vi "P116x1ch_WriteManual.vi"(5 "P116x1ch":T1, 7 "Decimales":T3=1 items=["0"=1, "1"=10, "2"=100], 8 "error in (no error)":errorcluster, 9 "RateSP":T2, 10 "NuevoSP":T2, 11 "Comunicaciones":T4={"Eurotherm"="ASRL6::INSTR", "CDT"=FALSE, "Agilent"="ASRL6::INSTR", "AGL"=FALSE, "#dec"=1} {"#dec" items=["1"=1, "1"=10, "2"=100]}) -> (0 "error out":errorcluster, 1 "RateSP(C/min) 2":T2, 2 "NuevoSP(C) 2":T2)   [LabVIEW 2017]
uses:
  1xP116.ctl
  Typedefs/SECADO_comms--Cluster.ctl
  numDecimales--Enum.ctl
  P116x1ch.ctl
  Address.ctl
  Eurotherm_2023_Module.ctl
panel:
  out "PV":T2
  out "WorkingSP":T2
  out "TargetSP":T2
  in  "Cancel":bool
  in  "Write":bool
  out "Enable(T)":bool=TRUE
  out "VISA Promux":refnum<visa-resource-name>
  in  "Delay Time (s)":dbl=0.1
  # "Programando Eurotherm"
  # "C/min"
  # "C"
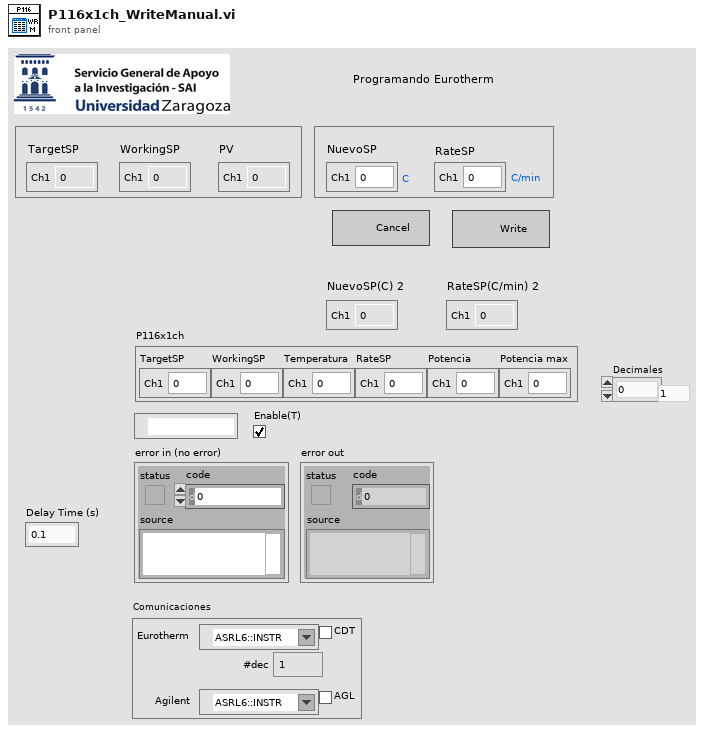
[diagram p1: front panel]
types:
  T1 = typedef "P116x1ch.ctl" = cluster{"TargetSP":T2, "WorkingSP":T2, "Temperatura":T2, "RateSP":T2, "Potencia":T2, "Potencia max":T2}
  T2 = typedef "1xP116.ctl" = cluster{"Ch1":dbl}
  T3 = typedef "numDecimales--Enum.ctl" = u16
  T4 = typedef "SECADO_comms--Cluster.ctl" = cluster{"Eurotherm":refnum<visa-resource-name>, "CDT":bool, "Agilent":refnum<visa-resource-name>, "AGL":bool, "#dec":T3}
  T5 = typedef "Eurotherm_2023_Module.ctl" = enum16{"Initialize", "Write setpoint", "Read data", "Write ramp rate", "Set constante proporcional", "Set constante integral", "Set constante diferencial", "Set ouput limit LOW", "Set ouput limit HIGH", "Shutdown"}
  T6 = typedef "Address.ctl" = enum16{"Add 1", "Add 2", "Add 3", "Add 4", "Add 5", "Add 6", "Add 10", "Add 11", "Add 12", "Add 13"}
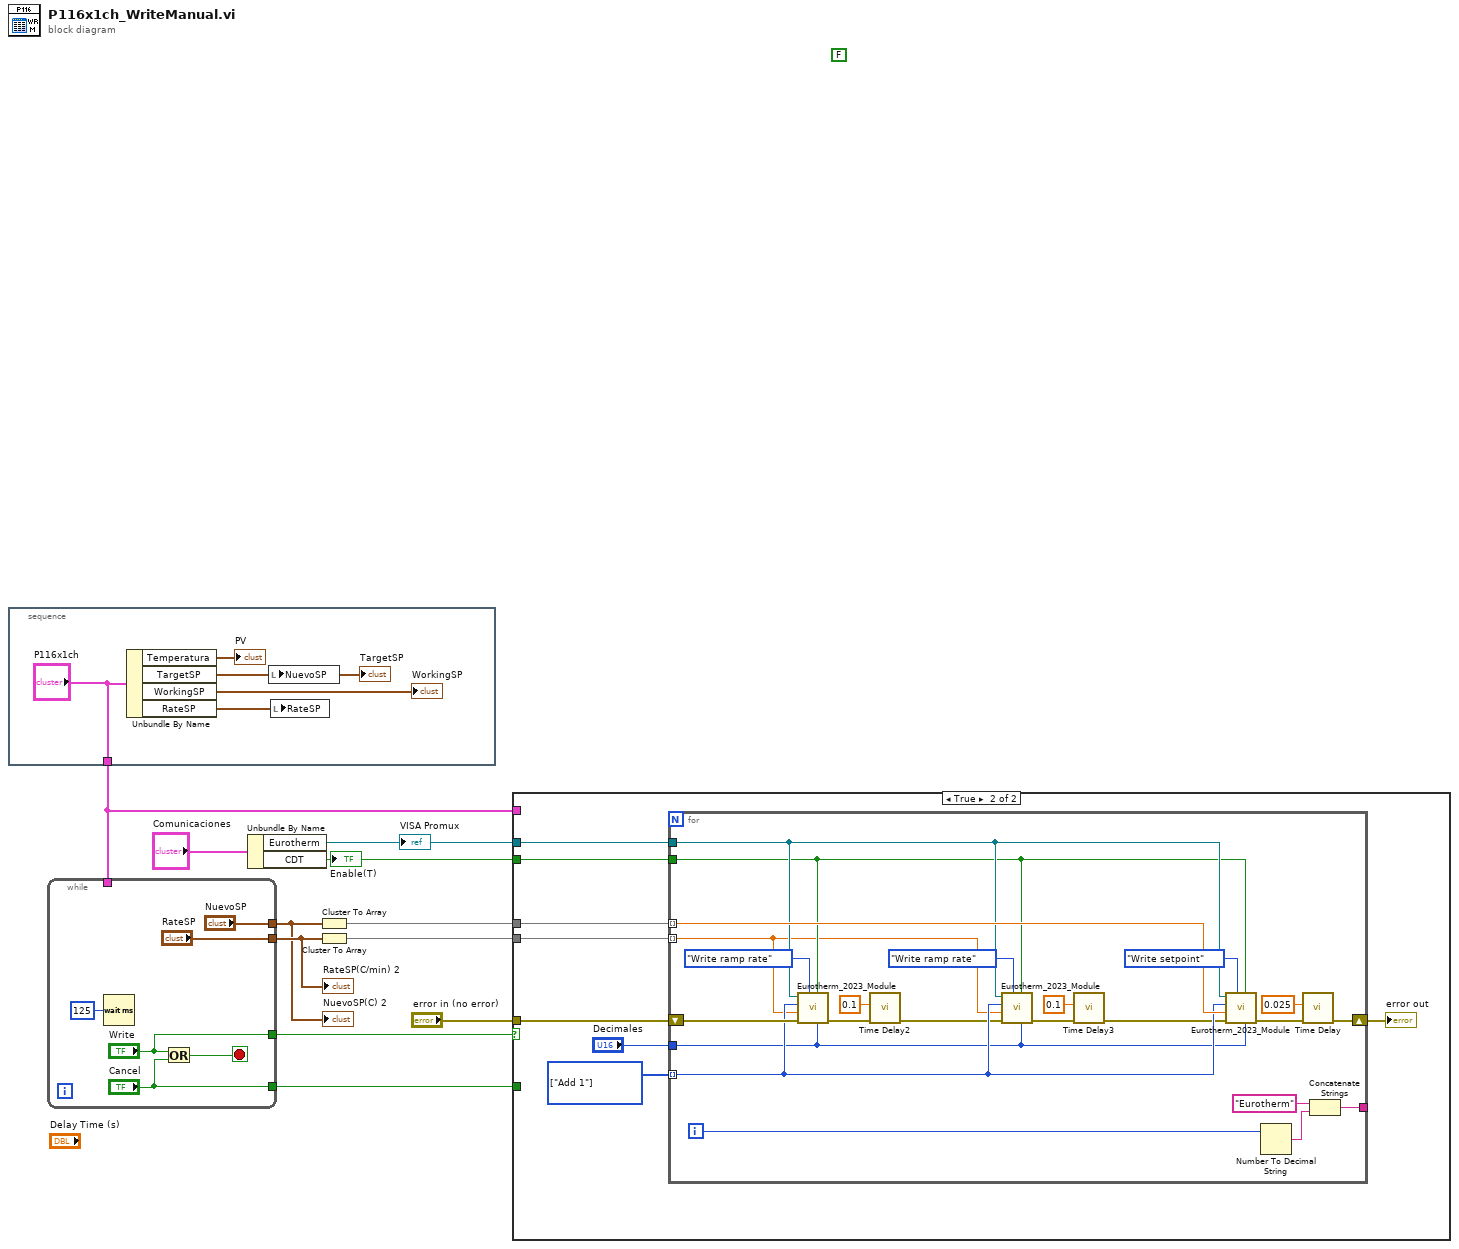
[diagram p0: block diagram]
diagram:
  (unwired) FALSE
  n1 = stacked-sequence {
    tunnel: ["P116x1ch"] -> w4
    frame #0 {
      n2 = Unbundle By Name("P116x1ch") -> ("Temperatura"=→"PV":T2, "TargetSP"=w14:T2, "WorkingSP"=→"WorkingSP":T2, "RateSP"=w13:T2)
      "TargetSP" <- w14
      n3 = local write "NuevoSP"(w14) -> ()
      n4 = local write "RateSP"(w13) -> ()
    }
  }
  n5 = while {
    tunnel: ["Cancel"] -> w10
    tunnel: ["NuevoSP"] -> w2
    tunnel: ["RateSP"] -> w3
    tunnel: ["Write"] -> w6
    tunnel: w4 -> [_]
    stop <- w17 stop-if-true
    n6 = Wait (ms)(milliseconds to wait=u32 125) -> ()  [unwired: 1 out]
    n7 = Or(x="Write", y="Cancel") -> (x .or. y?=w17:bool)
  }
  "NuevoSP(C) 2" <- w2
  "RateSP(C/min) 2" <- w3
  n8 = Unbundle By Name("Comunicaciones") -> ("Eurotherm"=w5:refnum<visa-resource-name>, "CDT"=w11:bool)
  "Enable(T)" <- w11
  "VISA Promux" <- w5
  n9 = Cluster To Array(cluster=w2) -> (array=w8:dbl[])
  n10 = Cluster To Array(cluster=w3) -> (array=w7:dbl[])
  n11 = case shown="True" w6 {
    tunnel: w11 -> [_ w29]
    tunnel: w10 -> [_ _]
    tunnel: "error in (no error)" -> [_ w27]
    tunnel: w8 -> [_ w25]
    tunnel: w7 -> [_ w26]
    tunnel: w5 -> [_ w30]
    tunnel: w4 -> [_ _]
    frame False {
    }
    frame True {
      w24 = T6[] [enum."Add 1"] items=["Add 1", "Add 2", "Add 3", "Add 4", "Add 5", "Add 6", "Add 10", "Add 11", "Add 12", "Add 13"]
      n12 = for {
        tunnel: w24 -> [w37] mode=indexing
        shift-right: [w44] -> w28
        shift-left: w27 -> [w48]
        tunnel: [w51] -> _
        tunnel: w25 -> [w46] mode=indexing
        tunnel: w26 -> [w32] mode=indexing
        tunnel: w30 -> [w34]
        tunnel: w29 -> [w33]
        tunnel: "Decimales" -> [w31]
        i -> [w43]
        n13 = call "Eurotherm_2023_Module.vi"("Decimales"=w31, "Eurotherm (T:Enable)"=w33, "Command"=Eurotherm_2023_Module."Write ramp rate", "error in (no error)"=w48, "Value"=w32, "Address"=w37, "VISA resource name"=w34) -> ("error out"=w42:errorcluster)  [unwired: 2 in, 2 out]
        n14 = call "Time Delay2"("error in (no error)"=w42, "Delay Time (s)"=0.1) -> ("error out"=w36:errorcluster)  [unwired: 9 in]
        n15 = call "Eurotherm_2023_Module.vi"("Decimales"=w31, "Eurotherm (T:Enable)"=w33, "Command"=Eurotherm_2023_Module."Write ramp rate", "error in (no error)"=w36, "Value"=w32, "Address"=w37, "VISA resource name"=w34) -> ("error out"=w39:errorcluster)  [unwired: 2 in, 2 out]
        n16 = call "Time Delay3"("error in (no error)"=w39, "Delay Time (s)"=0.1) -> ("error out"=w35:errorcluster)  [unwired: 9 in]
        n17 = call "Eurotherm_2023_Module.vi"("Decimales"=w31, "Eurotherm (T:Enable)"=w33, "Command"=Eurotherm_2023_Module."Write setpoint", "error in (no error)"=w35, "Value"=w46, "Address"=w37, "VISA resource name"=w34) -> ("error out"=w45:errorcluster)  [unwired: 2 in, 2 out]
        n18 = Number To Decimal String(number=w43) -> (decimal integer string=w52:string)  [unwired: 1 in]
        n19 = call "Time Delay"("error in (no error)"=w45, "Delay Time (s)"=0.025) -> ("error out"=w44:errorcluster)  [unwired: 9 in]
        n20 = Concatenate Strings("Eurotherm" ("error source (\" \")"), w52) -> (w51:string)
      }
      "error out" <- w28
    }
  }
